vi "TestMoveAnalysers.vi"() -> ()   [LabVIEW 2014]
panel:
  in  "STOP":bool
  out "Interrupts":bool[](array[boolean])
  out "Inputs":bool[](array[boolean])
  in  "Pulse Override":bool[](array[boolean])
  in  "State":bool[](array[boolean])
  in  "Steps/ second":i32
  # "P0.1"
  # "A1 Direction"
  # "A2 stepper"
  # "P0.2"
  # "A2 direction"
  # "P0.4"
  # "P0.5"
  # "P0.7"
  # "A1 Stepper"
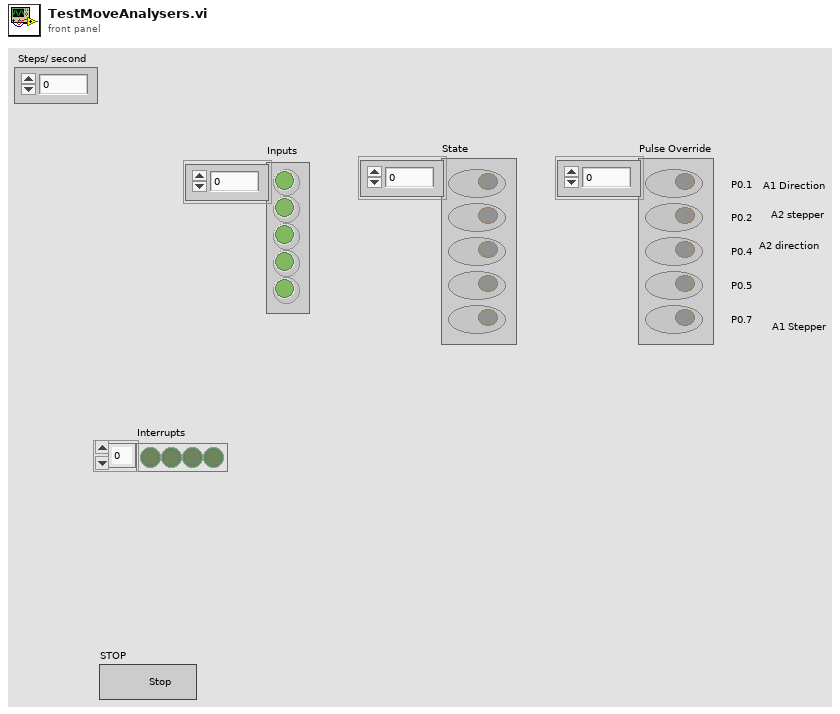
[diagram p1: front panel]
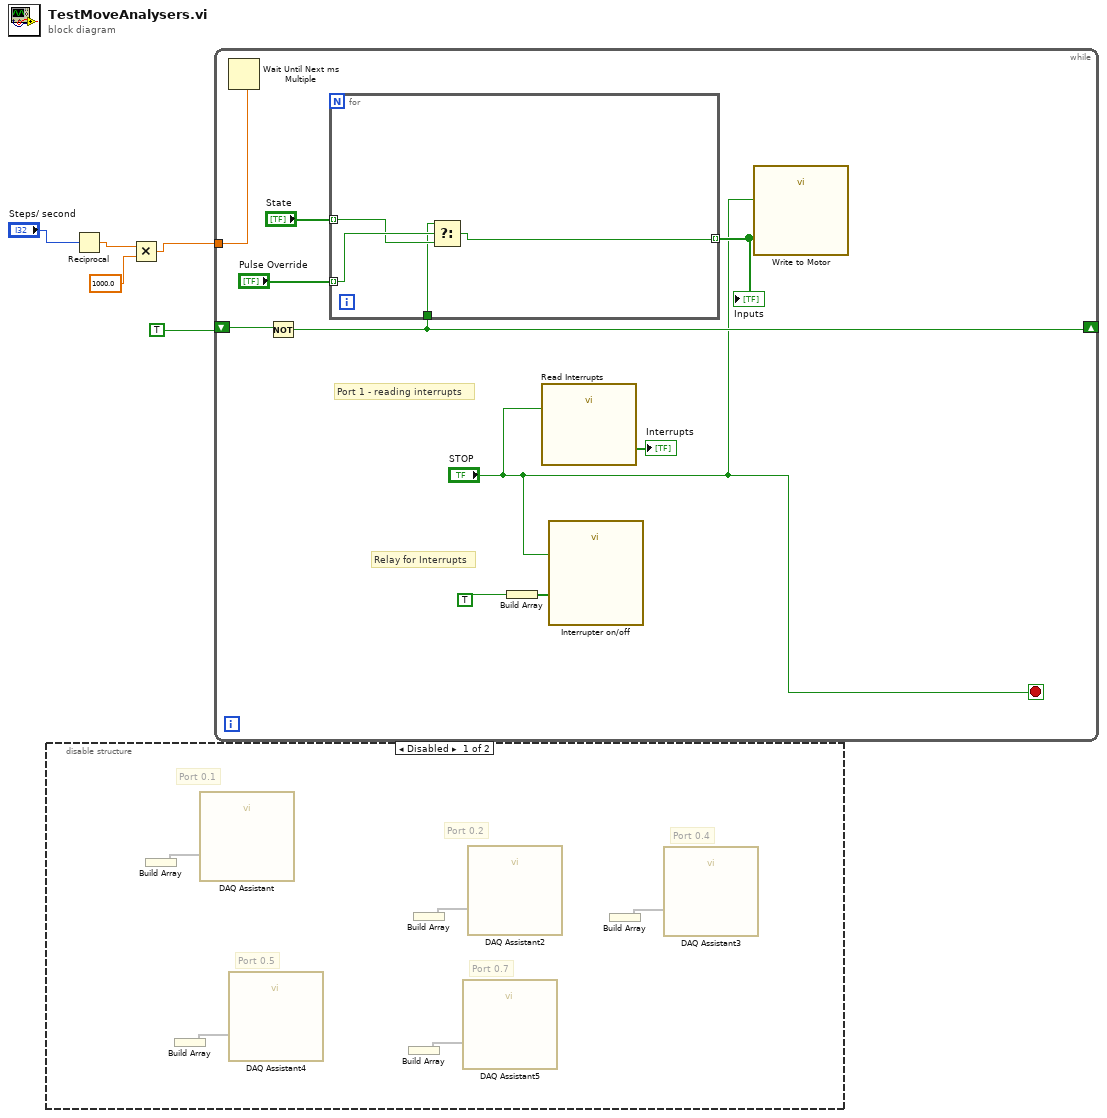
[diagram p0: block diagram]
diagram:
  n1 = disable-structure shown="Disabled" {
    frame Disabled {
      # "Port 0.1"
      # "Port 0.7"
      # "Port 0.5"
      # "Port 0.4"
      # "Port 0.2"
      n2 = Build Array() -> (w6:void[], w7:dbl)
      n3 = Build Array() -> (w9:void[])  [unwired: 1 in]
      n4 = call "DAQ Assistant"("data"=w6) -> ()  [unwired: 17 in, 2 out]
      n5 = call "DAQ Assistant4"("data"=w9) -> ()  [unwired: 17 in, 2 out]
      n6 = Build Array() -> (w8:void[])  [unwired: 1 in]
      n7 = Build Array() -> (w11:void[])  [unwired: 1 in]
      n8 = call "DAQ Assistant5"("data"=w8) -> ()  [unwired: 17 in, 2 out]
      n9 = call "DAQ Assistant2"("data"=w11) -> ()  [unwired: 17 in, 2 out]
      n10 = Build Array() -> (w10:void[])  [unwired: 1 in]
      n11 = call "DAQ Assistant3"("data"=w10) -> ()  [unwired: 17 in, 2 out]
    }
    frame Enabled {
    }
  }
  n12 = Reciprocal(x="Steps/ second") -> (1/x=w4:dbl)
  n13 = Multiply(x=w4, y=1000.0) -> (x*y=w2:dbl)
  n14 = while {
    tunnel: w2 -> [w21]
    shift-right: [w17] -> _
    shift-left: TRUE -> [w20]
    stop <- "STOP" stop-if-true
    # "Relay for Interrupts"
    # "Port 1 - reading interrupts"
    n15 = Wait Until Next ms Multiple(millisecond multiple=w21) -> ()  [unwired: 1 out]
    n16 = Not(x=w20) -> (.not. x?=w17:bool)
    n17 = for {
      tunnel: "State" -> [w24] mode=indexing
      tunnel: "Pulse Override" -> [w25] mode=indexing
      tunnel: w17 -> [w23]
      tunnel: [w22] -> w16 mode=indexing
      n18 = Select(t=w23, s=w25, f=w24) -> (s? t:f=w22:bool)
    }
    "Inputs" <- w16
    n19 = Build Array(TRUE ("Relay Switch")) -> (w13:bool[])
    n20 = call "Read Interrupts"("stop (T)"="STOP") -> ("data"=→"Interrupts":bool[])  [unwired: 16 in, 2 out]
    n21 = call "Interrupter on/off"("data"=w13, "stop (T)"="STOP") -> ()  [unwired: 16 in, 2 out]
    n22 = call "Write to Motor"("data"=w16, "stop (T)"="STOP") -> ()  [unwired: 16 in, 2 out]
  }
